vi "MFP3D Acquired Data.vi"() -> ()   [LabVIEW 2013]
uses:
  <vilib>/Platform/TimedLoop/XDataNode/timing_clust.ctl
  <vilib>/Platform/TimedLoop/XDataNode/nitl_modes.ctl
  <vilib>/Platform/TimedLoop/XDataNode/wakeup.ctl
  <vilib>/DAQmx/read.llb/DAQmx Read (Analog 1D DBL NChan 1Samp).vi
  subVIs/Driver Variables.vi
  <vilib>/DAQmx/create/channels.llb/DAQmx Create Channel (AI-Voltage-Basic).vi
  <vilib>/DAQmx/configure/timing.llb/DAQmx Timing (Sample Clock).vi
  <vilib>/DAQmx/miscellaneous.llb/DAQmx Fill In Error Info.vi
  <vilib>/Platform/TimedLoop/XDataNode/XDataNode.xnode
  <vilib>/Platform/TimedLoop/XDataNode/XDNodeRunTimeDep.lvlib
panel:
  in  "Reset Graphs":bool
  in  "Data Queue":refnum<queue>
  in  "Skip Back Button":bool
  in  "FF Speed":dbl=2.0
  in  "Progress":dbl(slide)=0.002 scale=0.0..1435.0
  in  "Seek Forward Button":bool
  in  "Media Stop Button":bool
  in  "Play Button":bool
  in  "Tabs":T1(tab)
  in  "Lockin Information":T2={"SR7265 Sensitivity (A)"=5e-07, "Excitation Voltage (V)"=0.1, "SR810 Sensitivity (A)"=0.1, "Femto Gain (V/A)"=1.0, "Frequency (Hz)"=27.0}
  in  "Channel 1 (z, x, y, defl, Vtip, 4t I, 4t V)":tag="Dev1/ai0:5"
  in  "TDMS File Name":string="SA02821"
  in  "TDMS Output Folder":path=path "P:/users1/Yuhe/cypher tdms"
  out "TDMS Path Result":path
  in  "View Data After?":bool
  out "Z Value":cluster{"Y":dbl[], "Y":dbl[]}[](graph)
  out "X Position":cluster{"Y":dbl[], "Y":dbl[]}[](graph)
  out "Y Position":cluster{"Y":dbl[], "Y":dbl[]}[](graph)
  out "Tip Deflection":cluster{"Y":dbl[], "Y":dbl[]}[](graph)
  out "Tip Voltage":cluster{"Y":dbl[], "Y":dbl[]}[](graph)
  out "2-Terminal Conductance":cluster{"Y":dbl[], "Y":dbl[]}[](graph)
  out "2-Terminal Resistance":cluster{"Y":dbl[], "Y":dbl[]}[](graph)
  out "4-Terminal Conductance":cluster{"Y":dbl[], "Y":dbl[]}[](graph)
  out "4-Terminal Resistance":cluster{"Y":dbl[], "Y":dbl[]}[](graph)
  in  "Background Image":refnum<vi>
  in  "Inkscape File (.svg)":refnum<vi>
  in  "Run":refnum<vi>
  in  "Abort":refnum<vi>
  in  "Lithography Data":T3(array[cluster])
  # "FUTURE: will be used for TDMS playback"
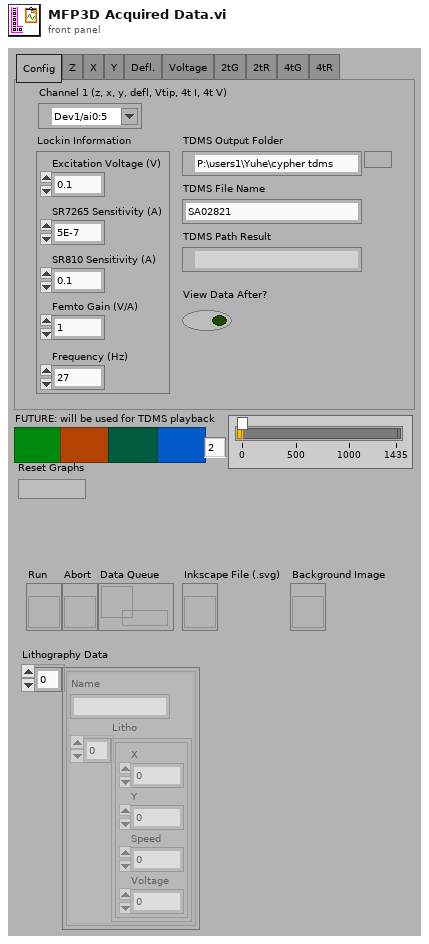
[diagram p1: front panel]
types:
  T1 = enum32{"Config", "Z", "X", "Y", "Defl.", "Voltage", "2tG", "2tR", "4tG", "4tR"}
  T2 = cluster{"SR7265 Sensitivity (A)":dbl, "Excitation Voltage (V)":dbl, "SR810 Sensitivity (A)":dbl, "Femto Gain (V/A)":dbl, "Frequency (Hz)":dbl}
  T3 = cluster{"Name":string, "Litho":cluster{"X":dbl, "Y":dbl, "Speed":dbl, "Voltage":dbl}[]}[]
  T4 = typedef "XDNodeRunTimeDep.lvlib/timing_clust.ctl" = cluster{"Expected End [f-1]":u64, "Actual End [f-1]":u64, "Finished Late? [f-1]":bool, "Expected End [i-1]":u64, "Actual End [i-1]":u64, "Finished Late? [i-1]":bool, "Expected Start [i]":u64, "Actual Start [i]":u64, "Expected Start [f]":u64, "Actual Start [f]":u64, "Source Name":string, "Structure Name":string, "Period":i64, "Deadline":i64, "Offset":i64, "Start":i64, "Priority":i32, "Timeout":i32, "Mode":T5, "Wakeup Reason":T6, "Error":errorcluster, "Source Type":string, "Secondary Source Type":string, "Global End Time":u64, "Global Start Time":u64, "Frame Duration":u64, "Iteration Duration":u64, "Assigned CPU":i32, "I/O Scan Engine Mode":u32}
  T5 = typedef "XDNodeRunTimeDep.lvlib/nitl_modes.ctl" = enum32{"No Change", "Process missed periods, maintain original phase", "Discard missed periods, maintain original phase", "Process missed periods, ignore original phase", "Discard missed periods, ignore original phase"}
  T6 = typedef "XDNodeRunTimeDep.lvlib/wakeup.ctl" = enum32{"Normal", "Aborted", "Asynchronous wakeup", "Timing source error", "Timed loop error", "Timeout"}
  T7 = cluster{"Result":dbl, "Result":dbl, "Result":dbl, "Result":dbl, "Result":dbl, "Result":dbl}
  T8 = cluster{"SR7265 Sensitivity (A)":dbl, "Excitation Voltage (V)":dbl, "Femto Gain (V/A)":dbl, "SR810 Sensitivity (A)":dbl}
  T9 = cluster{"x":dbl, "y":dbl, "Voltage":dbl, "Voltage":dbl}
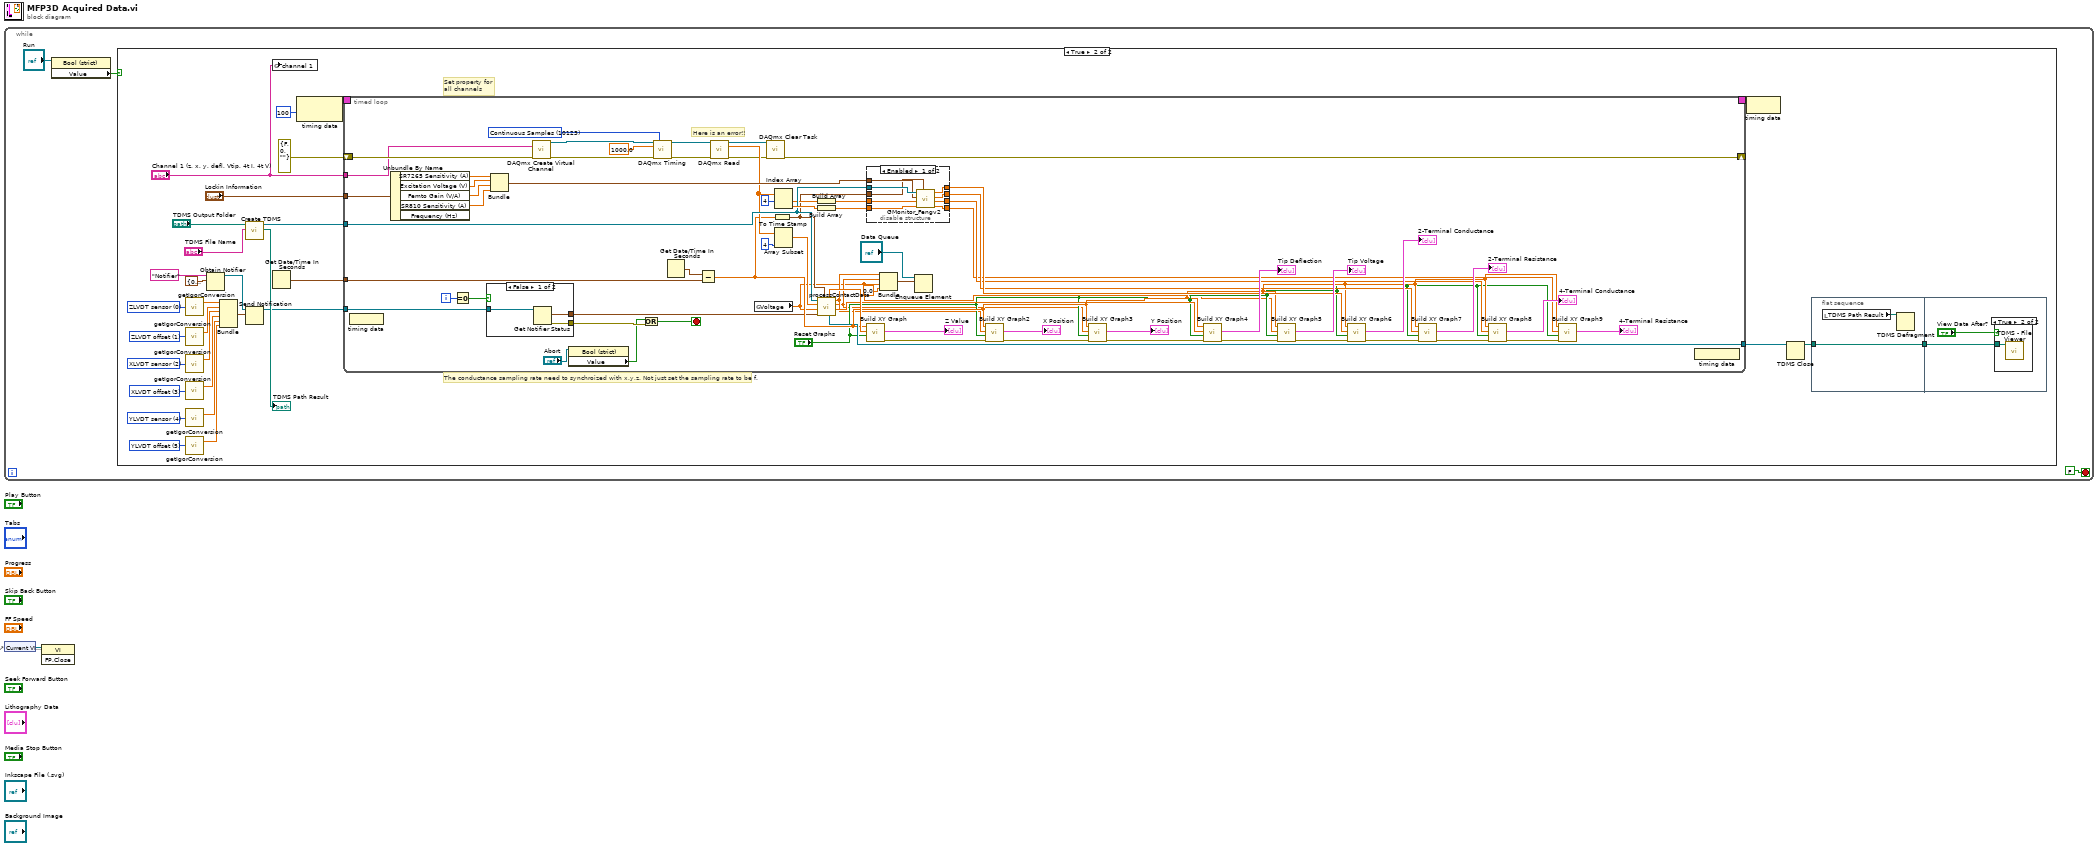
[diagram p0: block diagram]
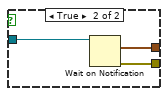
[diagram p5: hidden frame]
diagram:
  n1 = while {
    stop <- FALSE stop-if-true
    n2 = property class="Bool (strict)"(reference="Run") -> ("Value"=w3:bool)  [unwired: 1 in, 2 out]
    n3 = case shown="True" w3 {
      frame False {
      }
      frame True {
        w16 = 5 items=["ZLVDT sensor", "ZLVDT offset", "XLVDT sensor", "XLVDT offset", "YLVDT sensor", "YLVDT offset", "DEFL"] ("index")
        w17 = 4 items=["ZLVDT sensor", "ZLVDT offset", "XLVDT sensor", "XLVDT offset", "YLVDT sensor", "YLVDT offset", "DEFL"] ("index")
        w18 = 3 items=["ZLVDT sensor", "ZLVDT offset", "XLVDT sensor", "XLVDT offset", "YLVDT sensor", "YLVDT offset", "DEFL"] ("index")
        w19 = 2 items=["ZLVDT sensor", "ZLVDT offset", "XLVDT sensor", "XLVDT offset", "YLVDT sensor", "YLVDT offset", "DEFL"] ("index")
        w20 = 1 items=["ZLVDT sensor", "ZLVDT offset", "XLVDT sensor", "XLVDT offset", "YLVDT sensor", "YLVDT offset", "DEFL"] ("index")
        w21 = 0 items=["ZLVDT sensor", "ZLVDT offset", "XLVDT sensor", "XLVDT offset", "YLVDT sensor", "YLVDT offset", "DEFL"] ("index")
        # "Set property for \nall channels"
        # "The conductance sampling rate need to synchroized with x,y,z. Not just set the sampling rate to be f."
        n4 = call "getIgorConversion.vi"("index"=w21) -> ("Result"=w15:dbl)  [unwired: 1 out]
        n5 = call "getIgorConversion.vi"("index"=w20) -> ("Result"=w14:dbl)  [unwired: 1 out]
        n6 = call "getIgorConversion.vi"("index"=w19) -> ("Result"=w13:dbl)  [unwired: 1 out]
        n7 = call "getIgorConversion.vi"("index"=w18) -> ("Result"=w12:dbl)  [unwired: 1 out]
        n8 = call "getIgorConversion.vi"("index"=w17) -> ("Result"=w11:dbl)  [unwired: 1 out]
        n9 = call "getIgorConversion.vi"("index"=w16) -> ("Result"=w10:dbl)  [unwired: 1 out]
        n10 = Obtain Notifier(name (unnamed)="Notifier", notification data type=cluster{dbl, dbl, dbl, dbl, dbl, dbl} {0.0, 0.0, 0.0, 0.0, 0.0, 0.0}) -> (notifier out=w8:refnum<notifier>)  [unwired: 2 in, 2 out]
        n11 = Bundle("Result"=w15, "Result"=w14, "Result"=w13, "Result"=w12, "Result"=w11, "Result"=w10) -> (w9:T7)  [unwired: 1 in]
        n12 = call "Create TDMS.vi"("TDMS File Name"="TDMS File Name", "TDMS Output Folder"="TDMS Output Folder") -> ("modified path"=→"TDMS Path Result":path, "Refnum out"=w24:refnum<k34>)  [unwired: 8 in]
        n13 = Send Notification(notification=w9, notifier=w8) -> (notifier out=w6:refnum<notifier>)  [unwired: 1 in, 1 out]
        n14 = global write "Driver Variables.vi" "channel 1"("Channel 1 (z, x, y, defl, Vtip, 4t I, 4t V)") -> ()
        n15 = Get Date/Time In Seconds() -> (seconds since 1Jan1904=w26:timestamp)
        n16 = node-c288(100) -> (w35:T4)
        n17 = timed-loop {
          timing: w35 -> [_]
          timing-out: [_] -> w34
          tunnel: w6 -> [w107]
          tunnel: w24 -> [w102]
          shift-right: [w64] -> _
          shift-left: errorcluster {"status"=FALSE, "code"=0, "source"=""} ("error out") -> [w58]
          tunnel: "Lockin Information" -> [w101]
          tunnel: [w103] -> w28
          tunnel: w26 -> [w95]
          tunnel: "Channel 1 (z, x, y, defl, Vtip, 4t I, 4t V)" -> [w55]
          i -> [w109]
          stop <- w48 stop-if-true
          w62 = 10123 items=["Finite Samples"=10178, "Continuous Samples"=10123, "Hardware Timed Single Point"=12522] ("sample mode")
          # "Here is an error!!"
          n18 = node-c288() -> ()  [unwired: 1 in]
          n19 = Unbundle By Name(w101) -> ("SR7265 Sensitivity (A)"=w96:dbl, "Excitation Voltage (V)"=w100:dbl, "Femto Gain (V/A)"=w99:dbl, "SR810 Sensitivity (A)"=w98:dbl)  [unwired: 1 out]
          n20 = Equal To 0?(x=w109) -> (x = 0?=w108:bool)
          n21 = case shown="False" w108 {
            tunnel: w107 -> [w121 w124]
            tunnel: [w120 w123] -> w50
            tunnel: [w119 w122] -> w52
            frame False {
              n22 = Get Notifier Status(notifier=w121) -> (current notification=w119:cluster{dbl, dbl, dbl, dbl, dbl, dbl}, error out=w120:errorcluster)  [unwired: 1 in, 3 out]
            }
            frame True {
              n23 = Wait on Notification(notifier=w124) -> (notification=w122:cluster{dbl, dbl, dbl, dbl, dbl, dbl}, error out=w123:errorcluster)  [unwired: 3 in, 2 out]
            }
          }
          n24 = Bundle("SR7265 Sensitivity (A)"=w96, "Excitation Voltage (V)"=w100, "Femto Gain (V/A)"=w99, "SR810 Sensitivity (A)"=w98) -> (w97:T8)  [unwired: 1 in]
          n25 = call-poly <vilib>:"DAQmx Create Virtual Channel.vi"("physical channels"=w55, "error in"=w58) -> ("task out"=w61:refnum<k21>, "error out"=w60:errorcluster)  [unwired: 12 in]
          n26 = property class="Bool (strict)"(reference="Abort") -> ("Value"=w49:bool)  [unwired: 1 in, 2 out]
          n27 = Or(x=w49, y=w50) -> (x .or. y?=w48:bool)
          n28 = call-poly <vilib>:"DAQmx Timing.vi"("task/channels in"=w61, "sample mode"=w62, "rate"=1000.0, "error in"=w60) -> ("task out"=w59:refnum<k21>, "error out"=w57:errorcluster)  [unwired: 10 in]
          n29 = Get Date/Time In Seconds() -> (seconds since 1Jan1904=w92:timestamp)
          n30 = Subtract(x=w92, y=w95) -> (x-y=w54:dbl)
          n31 = call-poly <vilib>:"DAQmx Read.vi"("task/channels in"=w59, "error in"=w57) -> ("task out"=w56:refnum<k21>, "data"=w66:dbl[], "error out"=w65:errorcluster)  [unwired: 11 in]
          n32 = global read "Driver Variables.vi" "Voltage"() -> (w44:dbl)
          n33 = call <vilib>:"DAQmx Clear Task.vi"("task in"=w56, "error in"=w65) -> ("error out"=w64:errorcluster)  [unwired: 13 in]
          n34 = To Time Stamp(1:w54) -> (0:w53:timestamp)
          n35 = Index Array(array=w66, index #1=4) -> (element #1=w78:dbl, element #2=w105:dbl)  [unwired: 1 in]
          n36 = Array Subset(array=w66, length=4) -> (w67:dbl[])  [unwired: 1 in]
          n37 = Build Array(w78) -> (w77:dbl[])
          n38 = Build Array(w105) -> (w104:dbl[])
          n39 = call "processContactData.vi"("tdms file"=w102, "data"=w67, "tip voltage"=w44, "lvdt"=w52, "time stamp"=w53) -> ("z"=w93:dbl, "tdms file out"=w103:refnum<k34>, "x"=w46:dbl, "y"=w45:dbl, "deflection"=w88:dbl)  [unwired: 1 out]
          n40 = disable-structure shown="Enabled" {
            disable-tunnel: w104 -> [w118 _]
            disable-tunnel: w102 -> [w117 _]
            disable-tunnel: w97 -> [w116 _]
            disable-tunnel: w53 -> [w115 _]
            disable-tunnel: [w114 _] -> w85
            disable-tunnel: [w113 _] -> w83
            disable-tunnel: [w112 _] -> w80
            disable-tunnel: [w111 _] -> w79
            disable-tunnel: w77 -> [w110 _]
            frame Enabled {
              n41 = call "GMonitor_Fengv2.vi"("Time Stamp"=w115, "v1"=w118, "v0"=w110, "lockin information"=w116, "tdms file"=w117) -> ("FtR"=w111:dbl, "FtG"=w112:dbl, "TtR"=w113:dbl, "TtG"=w114:dbl)  [unwired: 1 out]
            }
            frame Disabled {
            }
          }
          n42 = call "Build XY Graph"("Reset"="Reset Graphs", "Y Input"=w93, "X Input"=w54) -> ("error out"=w76:errorcluster, "XY Graph"=→"Z Value":cluster{"X":dbl[], "Y":dbl[]}[])  [unwired: 7 in]
          n43 = Bundle("x"=w46, "y"=w45, "Voltage"=w44, "Voltage"=0.0) -> (w42:T9)  [unwired: 1 in]
          n44 = Enqueue Element(queue="Data Queue", element=w42) -> ()  [unwired: 2 in, 3 out]
          n45 = call "Build XY Graph2"("error in (no error)"=w76, "Reset"="Reset Graphs", "Y Input"=w46, "X Input"=w54) -> ("error out"=w75:errorcluster, "XY Graph"=→"X Position":cluster{"X":dbl[], "Y":dbl[]}[])  [unwired: 6 in]
          n46 = call "Build XY Graph3"("error in (no error)"=w75, "Reset"="Reset Graphs", "Y Input"=w45, "X Input"=w54) -> ("error out"=w74:errorcluster, "XY Graph"=→"Y Position":cluster{"X":dbl[], "Y":dbl[]}[])  [unwired: 6 in]
          n47 = call "Build XY Graph4"("error in (no error)"=w74, "Reset"="Reset Graphs", "Y Input"=w88, "X Input"=w54) -> ("error out"=w73:errorcluster, "XY Graph"=→"Tip Deflection":cluster{"X":dbl[], "Y":dbl[]}[])  [unwired: 6 in]
          n48 = call "Build XY Graph5"("error in (no error)"=w73, "Reset"="Reset Graphs", "Y Input"=w44, "X Input"=w54) -> ("error out"=w72:errorcluster, "XY Graph"=→"Tip Voltage":cluster{"X":dbl[], "Y":dbl[]}[])  [unwired: 6 in]
          n49 = call "Build XY Graph6"("error in (no error)"=w72, "Reset"="Reset Graphs", "Y Input"=w85, "X Input"=w54) -> ("error out"=w71:errorcluster, "XY Graph"=→"2-Terminal Conductance":cluster{"X":dbl[], "Y":dbl[]}[])  [unwired: 6 in]
          n50 = call "Build XY Graph7"("error in (no error)"=w71, "Reset"="Reset Graphs", "Y Input"=w83, "X Input"=w54) -> ("error out"=w70:errorcluster, "XY Graph"=→"2-Terminal Resistance":cluster{"X":dbl[], "Y":dbl[]}[])  [unwired: 6 in]
          n51 = call "Build XY Graph8"("error in (no error)"=w70, "Reset"="Reset Graphs", "Y Input"=w80, "X Input"=w54) -> ("error out"=w69:errorcluster, "XY Graph"=→"4-Terminal Conductance":cluster{"X":dbl[], "Y":dbl[]}[])  [unwired: 6 in]
          n52 = call "Build XY Graph9"("error in (no error)"=w69, "Reset"="Reset Graphs", "Y Input"=w79, "X Input"=w54) -> ("XY Graph"=→"4-Terminal Resistance":cluster{"X":dbl[], "Y":dbl[]}[])  [unwired: 6 in, 1 out]
          n53 = node-c288() -> ()  [unwired: 1 out]
        }
        n54 = node-c288(w34) -> ()
        n55 = TDMS Close(11:w28) -> (3:w27:path)  [unwired: 1 in, 1 out]
        n56 = flat-sequence {
          tunnel: w27 -> [w37]
          tunnel: [w37] -> w33
          tunnel: w33 -> [w39]
          frame #0 {
            n57 = local read "TDMS Path Result"() -> (w36:path)
            n58 = TDMS Defragment(7:w36) -> ()  [unwired: 1 in, 1 out]
          }
          frame #1 {
            n59 = case shown="True" "View Data After?" {
              tunnel: w39 -> [_ w40]
              frame False {
              }
              frame True {
                n60 = call <vilib>:"TDMS - File Viewer.vi"("file path"=w40) -> ()  [unwired: 5 in, 2 out]
              }
            }
          }
        }
      }
    }
  }
  n61 = control-ref of="Current VI Reference"() -> (w1:refnum<vi>)
  n62 = invoke class="VI" method="FP.Close"(reference=w1) -> ()  [unwired: 2 in, 3 out]
